vi "Get Multiple Wheels in Steering Frame by Name.vi"(8 "error in (no error)":errorcluster, 10 "wheel names":string[](array[string]), 11 "steering frame in":refnum<class "NI_Robotics_Steering Frame.lvclass">) -> (0 "error out":errorcluster, 1 "found?":bool[](array[boolean]), 2 "wheels":refnum<class "NI_Robotics_Wheel.lvclass">[](array[class]), 3 "steering frame out":refnum<class "NI_Robotics_Steering Frame.lvclass">, 4 "frame angles (rad)":dbl[](array[numeric]), 5 "y positions":dbl[](array[numeric]), 7 "x positions":dbl[](array[numeric]))   [LabVIEW 2017, in "NI_Robotics_Steering Frame.lvclass"]
doc: "Returns the wheels you specify in <B>steering frame in</B> and properties of those wheels. You must manually select the polymorphic instance to use."
uses:
  <vilib>/robotics/Steering/Steering Frame/NI_Robotics_Steering Frame.lvclass
  <vilib>/robotics/Steering/Wheel/NI_Robotics_Wheel.lvclass
  <vilib>/robotics/Steering/Steering Frame/NI_Robotics_Steering Frame.lvclass/NI_Robotics_Steering Frame.ctl
  <vilib>/robotics/Steering/Wheel/NI_Robotics_Wheel.lvclass/NI_Robotics_Wheel.ctl
  <vilib>/robotics/Steering/Wheel/Get Wheel Name.vi
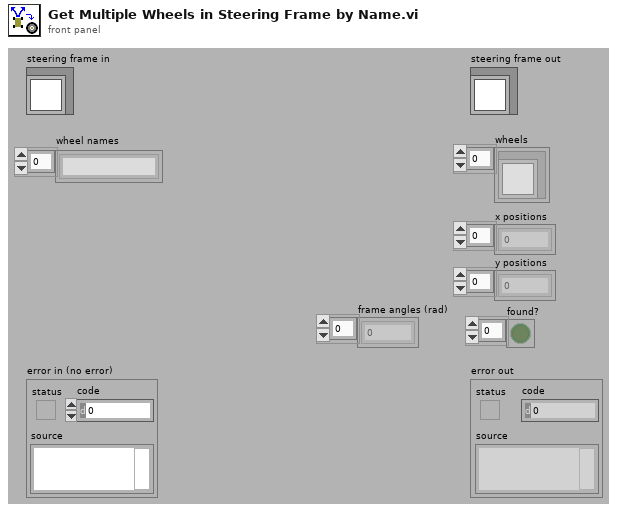
[diagram p1: front panel]
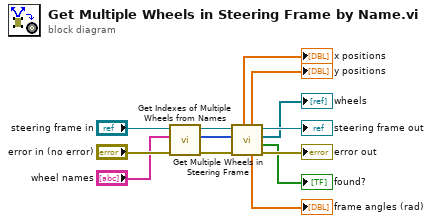
[diagram p0: block diagram]
diagram:
  n1 = call <vilib>:"Get Indexes of Multiple Wheels from Names.vi"("error in (no error)"="error in (no error)", "wheel names"="wheel names", "steering frame in"="steering frame in") -> ("error out"=w10:errorcluster, "indexes"=w11:i32[], "steering frame out"=w12:refnum<class "NI_Robotics_Steering Frame.lvclass">)  [unwired: 5 in, 1 out]
  n2 = call <vilib>:"Get Multiple Wheels in Steering Frame.vi"("error in (no error)"=w10, "wheel indexes"=w11, "steering frame in"=w12) -> ("error out"=→"error out":errorcluster, "found?"=→"found?":bool[], "wheels"=→"wheels":refnum<class "NI_Robotics_Wheel.lvclass">[], "steering frame out"=→"steering frame out":refnum<class "NI_Robotics_Steering Frame.lvclass">, "frame angles (rad)"=→"frame angles (rad)":dbl[], "y positions"=→"y positions":dbl[], "x positions"=→"x positions":dbl[])  [unwired: 2 in]
